vi "Document_AddParagraphCollection.vi"(8 "error in (no error)":errorcluster, 10 "ParagraphCollection":refnum<k24>, 11 "ooWriter in":refnum<class "ooWriter.lvclass">) -> (0 "error out":errorcluster, 3 "ooWriter out":refnum<class "ooWriter.lvclass">)   [LabVIEW 2009, in "ooWriter.lvclass"]
uses:
  ooWriter.lvclass
  C:/Projets/LAVAG/OpenOfficeRGT/AODL/DLLs/AODL.dll
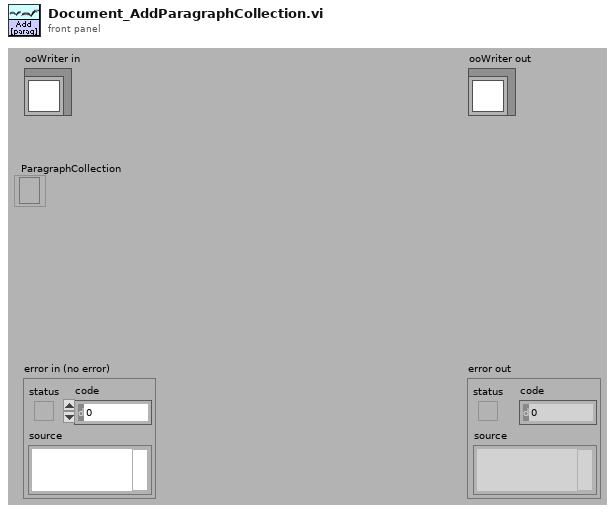
[diagram p1: front panel]
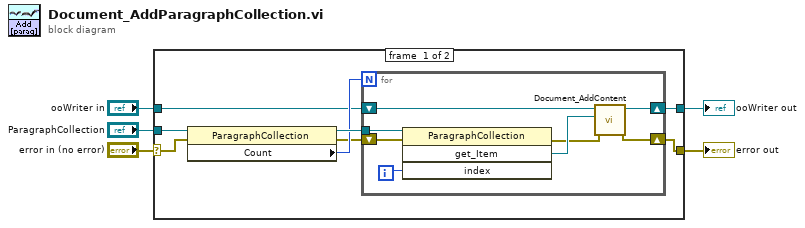
[diagram p0: block diagram]
diagram:
  n1 = case shown="No Error" "error in (no error)" {
    selector: "error in (no error)" -> [w7 w23]
    tunnel: [w6 w23] -> w4
    tunnel: [w9 w22] -> w2
    tunnel: "ooWriter in" -> [w10 w22]
    tunnel: "ParagraphCollection" -> [w13 _]
    frame #0 {
      n2 = property class="ParagraphCollection"(reference=w13, error in=w7) -> (reference out=w12:refnum<k24>, error out=w8:errorcluster, "Count"=w11:i32)
      n3 = for {
        N: w11 -> [_]
        tunnel: w12 -> [w21]
        shift-right: [w18] -> w9
        shift-left: w10 -> [w19]
        shift-right: [w14] -> w6
        shift-left: w8 -> [w16]
        i -> [w20]
        n4 = invoke class="ParagraphCollection" method="get_Item"(reference=w21, error in=w16, "index"=w20) -> (error out=w15:errorcluster, "get_Item"=w17:refnum<k24>)  [unwired: 1 in, 2 out]
        n5 = call-dynamic "Document_AddContent.vi"("error in (no error)"=w15, "Content"=w17, "ooWriter in"=w19) -> ("error out"=w14:errorcluster, "ooWriter out"=w18:refnum<class "ooWriter.lvclass">)  [unwired: 7 in]
      }
    }
    frame #1 {
    }
  }
  "error out" <- w4
  "ooWriter out" <- w2
